vi "PickNextMeasZ.vi"(8 "error in (no error)":errorcluster, 9 "warnings in":errorcluster, 10 "Log file":path=path "nologfile", 11 "Meas index":T1={"curr index"=0, "next index"=1, "num reps"=0, "allowed rep"=3, "SC count"=0, "SC interval"=20}) -> (0 "error out":errorcluster, 2 "new Meas index":T1={"curr index"=0, "next index"=1, "num reps"=0, "allowed rep"=3, "SC count"=0, "SC interval"=20})   [LabVIEW 2016]
doc: "This program selects the next set of intensity measurement conditions (measSetId) to be run. If an error or warning was found on the previous measurement, a dialog is displayed for a user to select which measurement to run next; if there is no response, the default is to repeat a measurement once, then move on. If no errors are found, the program checks for user interrupts. The next measurement is set to the user interrupt value if an interrupt is found, or if not, the next value in the input list is taken. The program also selects spot check measurements at a given interval."
panel:
  in  "Dialog sec":i32=60
  # "Program constants"
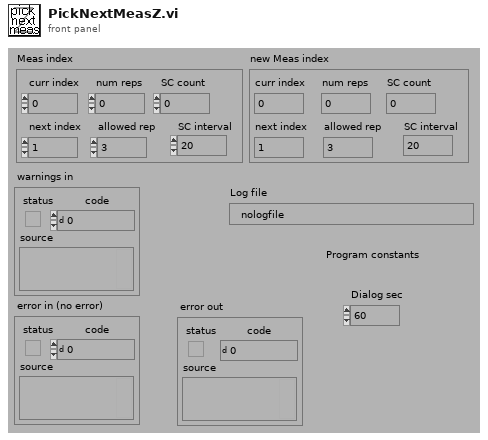
[diagram p1: front panel]
types:
  T1 = cluster{"curr index":u16, "next index":u16, "num reps":u16, "allowed rep":u16, "SC count":u16, "SC interval":u16}
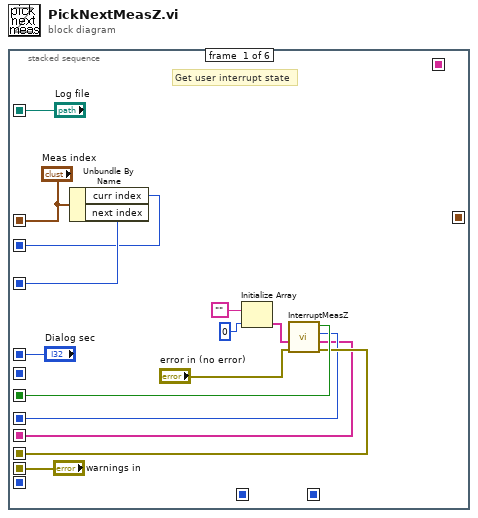
[diagram p0: block diagram]
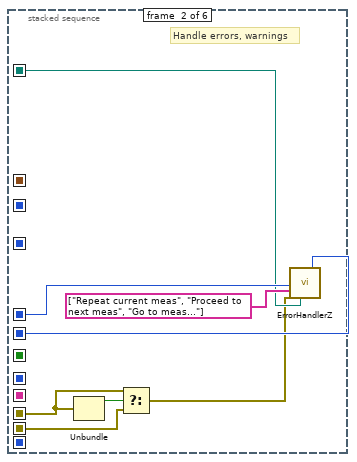
[diagram p2: hidden frame]
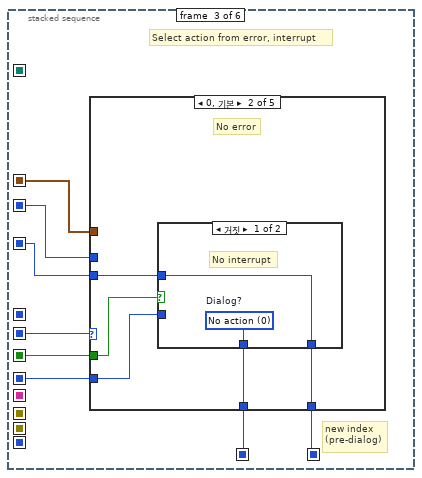
[diagram p3: hidden frame]
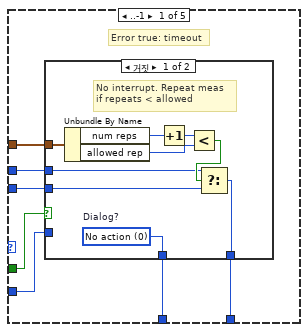
[diagram p4: hidden frame]
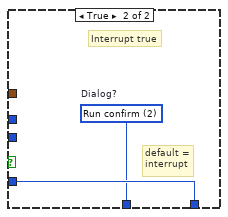
[diagram p5: hidden frame]
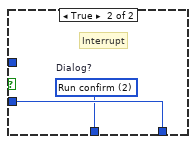
[diagram p6: hidden frame]
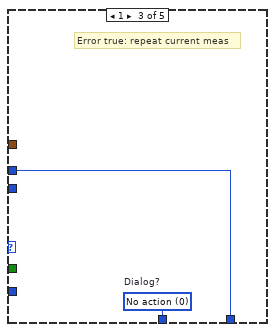
[diagram p7: hidden frame]
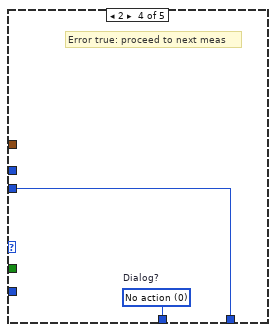
[diagram p8: hidden frame]
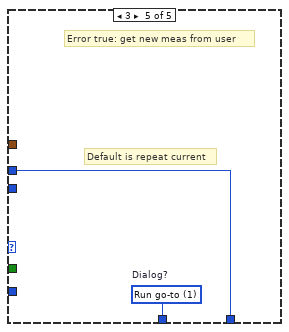
[diagram p9: hidden frame]
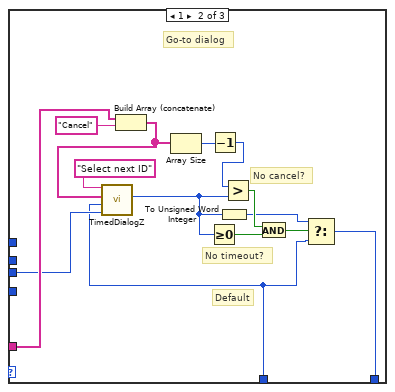
[diagram p11: hidden frame]
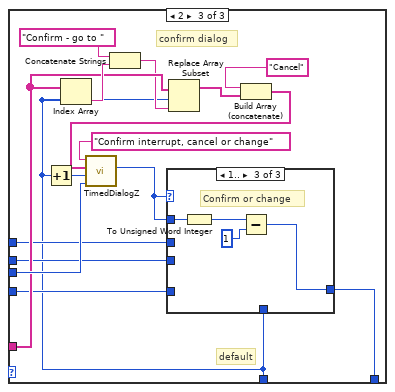
[diagram p12: hidden frame]
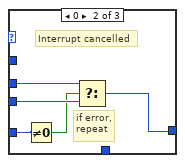
[diagram p14: hidden frame]
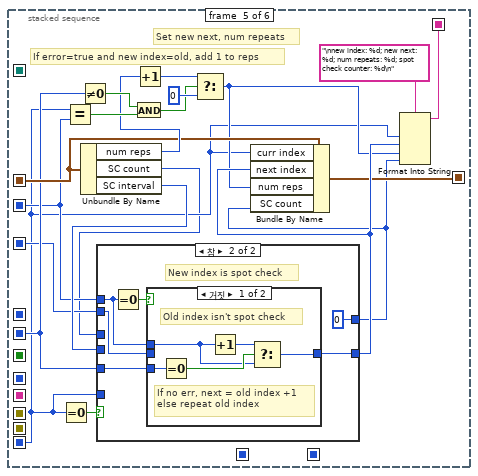
[diagram p15: hidden frame]
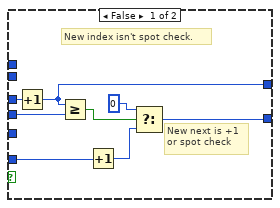
[diagram p16: hidden frame]
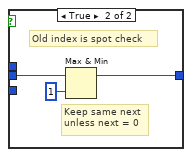
[diagram p17: hidden frame]
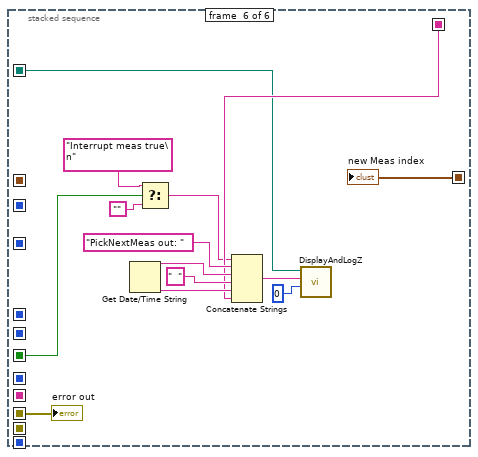
[diagram p18: hidden frame]
diagram:
  n1 = stacked-sequence {
    seq-local: [w14 _ _ _ _ _] -> [_ _ w29 _ _ w158]
    seq-local: [w12 _ _ _ _ _] -> [_ _ w27 _ _ _]
    seq-local: [w13 _ _ _ _ _] -> [_ w17 _ _ _ w155]
    seq-local: [_ w21 _ _ _ _] -> [_ _ w30 w67 w119 _]
    seq-local: [_ _ w28 _ _ _] -> [_ _ _ w69 _ _]
    seq-local: [w11 _ _ _ _ _] -> [_ _ _ w70 _ _]
    seq-local: [_ _ _ w68 _ _] -> [_ _ _ _ w116 _]
    seq-local: [_ _ w26 _ _ _] -> [_ _ _ w71 _ _]
    seq-local: [_ _ _ _ w125 _] -> [_ _ _ _ _ w162]
    seq-local: [w7 _ _ _ _ _] -> [_ _ w25 w65 w117 _]
    seq-local: [w6 _ _ _ _ _] -> [_ _ w24 w66 w118 _]
    seq-local: ["Meas index" _ _ _ _ _] -> [_ _ w23 _ w123 _]
    seq-local: ["Dialog sec" _ _ _ _ _] -> [_ w20 _ w64 _ _]
    seq-local: ["Log file" _ _ _ _ _] -> [_ w19 _ _ _ w161]
    seq-local: [_ _ _ _ w115 _] -> [_ _ _ _ _ w160]
    seq-local: ["warnings in" _ _ _ _ _] -> [_ w16 _ _ _ _]
    frame #0 {
      # "Get user interrupt state"
      n2 = Unbundle By Name("Meas index") -> ("curr index"=w6:u16, "next index"=w7:u16)
      n3 = Initialize Array("", 0 ("Dimension Size")) -> (w8:string[])
      n4 = call "InterruptMeasZ.vi"("error in (no error)"="error in (no error)", "meas_id"=w8) -> ("error out"=w13:errorcluster, "Select list out"=w11:string[], "new next index"=w12:u16, "Interrupt after meas"=w14:bool)  [unwired: 5 in, 1 out]
    }
    frame #1 {
      # "Handle errors, warnings"
      n5 = Unbundle(w17) -> ("status"=w18:bool)  [unwired: 2 out]
      n6 = Select(t=w17, s=w18, f=w16) -> (s? t:f=w15:errorcluster)
      n7 = call "ErrorHandlerZ.vi"("dialog sec (60)"=w20, "dialog prompts"=string[] ["Repeat current meas", "Proceed to next meas", "Go to meas..."], "error in (no error)"=w15, "Log file"=w19) -> ("selection/timeout (0)"=w21:i16)  [unwired: 10 in, 5 out]
    }
    frame #2 {
      # "new index\n(pre-dialog)"
      # "Select action from error, interrupt"
      n8 = case shown="0, 기본" w30 {
        tunnel: w29 -> [w37 w53 _ _ _]
        tunnel: [w36 w52 w59 w61 w62] -> w28
        tunnel: w27 -> [w35 w51 _ _ _]
        tunnel: w24 -> [w34 _ w59 _ w62]
        tunnel: w25 -> [w33 w50 _ w61 _]
        tunnel: [w32 w49 w58 w60 w63] -> w26
        tunnel: w23 -> [w31 _ _ _ _]
        frame ..-1 {
          # "Error true: timeout"
          n9 = case shown="거짓" w37 {
            tunnel: [w42 w48] -> w36
            tunnel: w35 -> [_ w48]
            tunnel: w34 -> [w44 _]
            tunnel: w33 -> [w43 _]
            tunnel: [w46 w47] -> w32
            tunnel: w31 -> [w41 _]
            frame False {
              w46 = u16 0 items=["No action", "Run go-to", "Run confirm"]  # Dialog?
              # "No interrupt. Repeat meas\nif repeats < allowed"
              n10 = Unbundle By Name(w41) -> ("num reps"=w39:u16, "allowed rep"=w40:u16)
              n11 = Increment(x=w39) -> (x+1=w38:u16)
              n12 = Less?(x=w38, y=w40) -> (x < y?=w45:bool)
              n13 = Select(t=w44, s=w45, f=w43) -> (s? t:f=w42:u16)
            }
            frame True {
              w47 = u16 2 items=["No action", "Run go-to", "Run confirm"]  # Dialog?
              # "default =\ninterrupt"
              # "Interrupt true"
            }
          }
        }
        frame 0, Default {
          # "No error"
          n14 = case shown="거짓" w53 {
            tunnel: [w55 w57] -> w52
            tunnel: w51 -> [_ w57]
            tunnel: w50 -> [w55 _]
            tunnel: [w54 w56] -> w49
            frame False {
              w54 = u16 0 items=["No action", "Run go-to", "Run confirm"]  # Dialog?
              # "No interrupt"
            }
            frame True {
              w56 = u16 2 items=["No action", "Run go-to", "Run confirm"]  # Dialog?
              # "Interrupt"
            }
          }
        }
        frame 1 {
          w58 = u16 0 items=["No action", "Run go-to", "Run confirm"]  # Dialog?
          # "Error true: repeat current meas"
        }
        frame 2 {
          w60 = u16 0 items=["No action", "Run go-to", "Run confirm"]  # Dialog?
          # "Error true: proceed to next meas"
        }
        frame 3 {
          w63 = u16 1 items=["No action", "Run go-to", "Run confirm"]  # Dialog?
          # "Default is repeat current"
          # "Error true: get new meas from user"
        }
      }
    }
    frame #3 {
      # "Dialog"
      n15 = case shown="0, 기본" w71 {
        tunnel: w64 -> [_ w80 w97]
        tunnel: w70 -> [_ w81 w94]
        tunnel: w69 -> [w72 w79 w87]
        tunnel: [w72 w75 w95] -> w68
        tunnel: w67 -> [_ _ w91]
        tunnel: w65 -> [_ _ w90]
        tunnel: w66 -> [_ _ w89]
        frame 0, Default {
          # "No dialog"
        }
        frame 1 {
          # "Default"
          # "No timeout?"
          # "No cancel?"
          # "Go-to dialog"
          n16 = Build Array (concatenate)(w81, "Cancel") -> (w84:string[])
          n17 = call "TimedDialogZ.vi"("dialog sec (60)"=w80, "options (0)"=w79, "option list"=w84, "Dialog text"="Select next ID") -> ("selection (timeout -1)"=w74:i32)  [unwired: 5 in]
          n18 = Array Size(array=w84) -> (size(s)=w83:i32)
          n19 = Greater Or Equal To 0?(x=w74) -> (x >= 0?=w78:bool)
          n20 = Decrement(x=w83) -> (x-1=w82:i32)
          n21 = To Unsigned Word Integer(number=w74) -> (unsigned 16bit integer=w73:u16)
          n22 = Greater?(x=w82, y=w74) -> (0:w77:bool)
          n23 = And(x=w77, y=w78) -> (x .and. y?=w76:bool)
          n24 = Select(t=w73, s=w76, f=w79) -> (s? t:f=w75:u16)
        }
        frame 2 {
          # "default"
          # "confirm dialog"
          n25 = Increment(x=w87) -> (x+1=w88:u16)
          n26 = Index Array(array=w94, index=w87) -> (element=w98:string)
          n27 = Concatenate Strings("Confirm - go to ", w98) -> (w93:string)
          n28 = Replace Array Subset(array=w94, new element=w93, index=w87) -> (w92:string[])
          n29 = Build Array (concatenate)("Cancel", w92) -> (w99:string[])
          n30 = call "TimedDialogZ.vi"("dialog sec (60)"=w97, "options (0)"=w88, "option list"=w99, "Dialog text"="Confirm interrupt, cancel or change") -> ("selection (timeout -1)"=w100:i32)  [unwired: 5 in]
          n31 = case shown="1.." w100 {
            tunnel: [w103 w104 w111] -> w95
            tunnel: w100 -> [_ _ w110]
            tunnel: w87 -> [w103 _ _]
            tunnel: w91 -> [_ w106 _]
            tunnel: w90 -> [_ w107 _]
            tunnel: w89 -> [_ w108 _]
            frame ..-1 {
              # "timeout: no change"
            }
            frame 0 {
              # "if error,\nrepeat"
              # "Interrupt cancelled"
              n32 = Not Equal To 0?(x=w106) -> (x != 0?=w105:bool)
              n33 = Select(t=w108, s=w105, f=w107) -> (s? t:f=w104:u16)
            }
            frame 1.. {
              # "Confirm or change"
              n34 = To Unsigned Word Integer(number=w110) -> (unsigned 16bit integer=w109:u16)
              n35 = Subtract(x=w109, y=u16 1) -> (x-y=w111:u16)
            }
          }
        }
      }
    }
    frame #4 {
      # "If error=true and new index=old, add 1 to reps"
      # "Set new next, num repeats"
      n36 = Equal To 0?(x=w116) -> (x = 0?=w132:bool)
      n37 = Equal?(x=w116, y=w118) -> (x = y?=w129:bool)
      n38 = Not Equal To 0?(x=w119) -> (x != 0?=w130:bool)
      n39 = Unbundle By Name(w123) -> ("num reps"=w124:u16, "SC count"=w114:u16, "SC interval"=w120:u16)
      n40 = case shown="참" w132 {
        tunnel: w118 -> [_ w143]
        tunnel: [w140 w145] -> w122
        tunnel: w114 -> [w134 _]
        tunnel: w120 -> [w139 _]
        tunnel: w119 -> [_ w146]
        tunnel: [w133 u16 0 ("Bundle Element")] -> w113
        tunnel: w117 -> [_ w141]
        tunnel: w116 -> [w137 _]
        frame False {
          # "New next is +1\nor spot check"
          # "New index isn't spot check."
          n41 = Increment(x=w134) -> (x+1=w133:u16)
          n42 = Greater Or Equal?(x=w133, y=w139) -> (x >= y?=w138:bool)
          n43 = Increment(x=w137) -> (x+1=w136:u16)
          n44 = Select(t=u16 0, s=w138, f=w136) -> (s? t:f=w140:u16)
        }
        frame True {
          # "New index is spot check"
          n45 = Equal To 0?(x=w143) -> (x = 0?=w142:bool)
          n46 = case shown="거짓" w142 {
            tunnel: w146 -> [w151 _]
            tunnel: w143 -> [w147 _]
            tunnel: [w148 w153] -> w145
            tunnel: w141 -> [_ w154]
            frame False {
              # "If no err, next = old index +1\nelse repeat old index"
              # "Old index isn't spot check"
              n47 = Equal To 0?(x=w151) -> (x = 0?=w150:bool)
              n48 = Increment(x=w147) -> (x+1=w149:u16)
              n49 = Select(t=w149, s=w150, f=w147) -> (s? t:f=w148:u16)
            }
            frame True {
              # "Keep same next\nunless next = 0"
              # "Old index is spot check"
              n50 = Max & Min(x=w154, y=u16 1) -> (max(x,y)=w153:u16)  [unwired: 1 out]
            }
          }
        }
      }
      n51 = And(x=w130, y=w129) -> (x .and. y?=w126:bool)
      n52 = Increment(x=w124) -> (x+1=w128:u16)
      n53 = Select(t=w128, s=w126, f=u16 0) -> (s? t:f=w121:u16)
      n54 = Bundle By Name(cluster=w123, "curr index"=w116, "next index"=w122, "num reps"=w121, "SC count"=w113) -> (w115:T1)
      n55 = Format Into String(format string="\nnew index: %d; new next: %d; num repeats: %d; spot check counter: %d\n", w116, w122, w121, w113) -> (resulting string=w125:string)  [unwired: 2 in, 1 out]
    }
    frame #5 {
      n56 = Get Date/Time String() -> (date string=w167:string, time string=w165:string)  [unwired: 3 in]
      n57 = Select(t="Interrupt meas true\n" ("Substring"), s=w158, f="") -> (s? t:f=w157:string)
      n58 = Concatenate Strings(w157, "PickNextMeas out: " ("Substring"), w167, "  ", w165, w162) -> (w164:string)
      n59 = call "DisplayAndLogZ.vi"("Log file"=w161, "message"=w164, "action (0: log+display)"=u16 0) -> ()  [unwired: 5 in, 1 out]
      "error out" <- w155
      "new Meas index" <- w160
    }
  }
